vi "Close.vi"(8 "error in (no error)":errorcluster, 11 "Controller in":refnum<class "Controller.lvclass">) -> (0 "error out":errorcluster, 3 "Controller out":refnum<class "Controller.lvclass">)   [LabVIEW 2019, in "Controller.lvclass"]
uses:
  Controller.lvclass
  Controller.lvclass/Controller.ctl
  Communication/Communication.lvclass
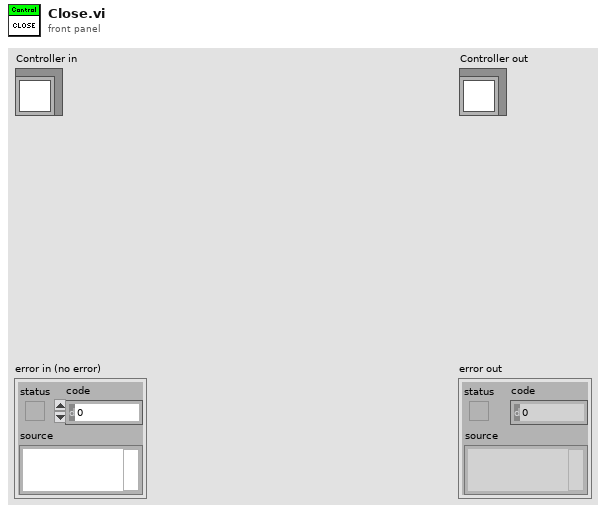
[diagram p1: front panel]
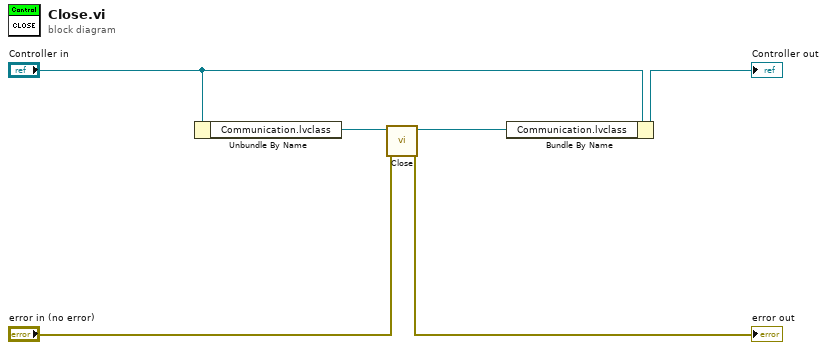
[diagram p0: block diagram]
diagram:
  n1 = Unbundle By Name("Controller in") -> ("Communication.lvclass"=w2:refnum<class "Communication.lvclass">)
  n2 = call "Close.vi"("error in (no error)"="error in (no error)", "Communication in"=w2) -> ("error out"=→"error out":errorcluster, "Communication out"=w1:refnum<class "Communication.lvclass">)  [unwired: 8 in]
  n3 = Bundle By Name(cluster="Controller in", "Communication.lvclass"=w1) -> (→"Controller out":refnum<class "Controller.lvclass">)
